vi "read last data.vi"(11 "Serial Port":refnum<visa-resource-name>) -> (2 "read string":string, 3 "Serial Port":refnum<visa-resource-name>)   [LabVIEW 2012]
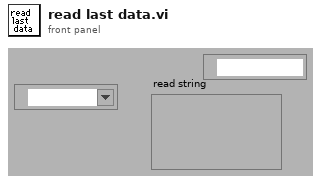
[diagram p1: front panel]
types:
  T1 = enum16{"Run Idle", "Pre Run", "SCC Pre Run 1", "SCC Pre Run 2", "SCC Run", "Run Active", "Report 1", "Report 2", "Run Disabled (from outside GC)"}
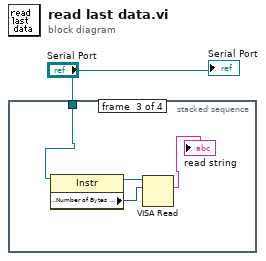
[diagram p0: block diagram]
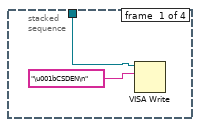
[diagram p2: hidden frame]
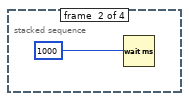
[diagram p3: hidden frame]
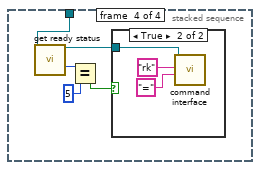
[diagram p4: hidden frame]
diagram:
  n1 = stacked-sequence {
    tunnel: "Serial Port" -> [w2 _ w6 w13]
    frame #0 {
      n2 = VISA Write(VISA resource name=w2, write buffer="\u001bCSDEN\n") -> ()  [unwired: 1 in, 3 out]
    }
    frame #1 {
      n3 = Wait (ms)(milliseconds to wait=1000) -> ()  [unwired: 1 out]
    }
    frame #2 {
      n4 = property class="Instr"(reference=w6) -> (reference out=w7:refnum<visa-resource-name>, "Serial Settings:Number of Bytes at Serial Port"=w8:u32)  [unwired: 1 in, 1 out]
      n5 = VISA Read(VISA resource name=w7, byte count=w8) -> (read buffer=→"read string":string)  [unwired: 1 in, 3 out]
    }
    frame #3 {
      n6 = call "get ready status.vi"("Serial Port"=w13) -> ("Serial Port"=w10:refnum<visa-resource-name>, "run status"=w12:T1)  [unwired: 10 in, 3 out]
      n7 = Equal?(x=w12, y=5) -> (x = y?=w9:bool)
      n8 = case shown="True" w9 {
        tunnel: w10 -> [_ w16]
        frame False {
        }
        frame True {
          n9 = call "command interface.vi"("Parameter"="=", "command"="rk", "Serial Port"=w16) -> ()  [unwired: 4 in, 4 out]
        }
      }
    }
  }
  "Serial Port" <- "Serial Port"
